vi "Edgertronic-pretrigger_buffer_fill_level.vi"(3 "error in (no error)":errorcluster, 5 "URL":string="192.168.1.101") -> (0 "error out":errorcluster, 1 "Pretrigger Buffer Fill Level:":T1={"Connection Information:"="", "Pretrigger Buffer Fill Level"="20140911165611"}, 2 "Fill Level":i32)   [LabVIEW 2015]
doc: "This VI returns the pretrigger buffer fill level."
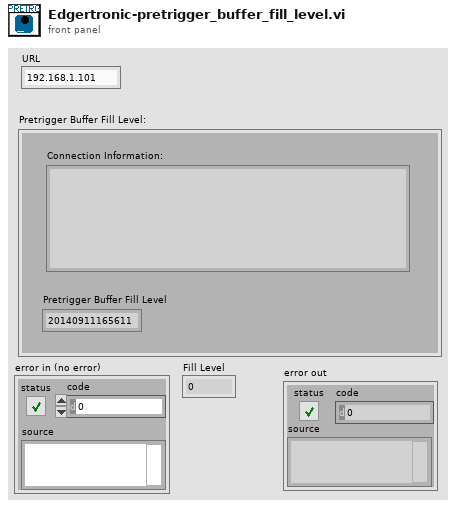
[diagram p1: front panel]
types:
  T1 = cluster{"Connection Information:":string, "Pretrigger Buffer Fill Level":string}
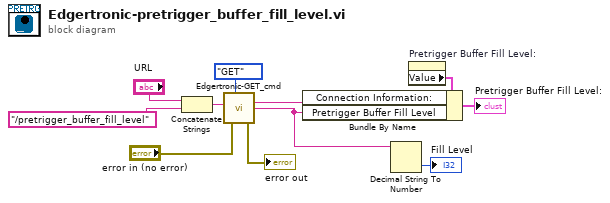
[diagram p0: block diagram]
diagram:
  n1 = Concatenate Strings("URL", "/pretrigger_buffer_fill_level" ("GET Cmd")) -> (w2:string)
  n2 = call "Edgertronic-GET_cmd.vi"("error in (no error)"="error in (no error)", "URL"=w2, "Type"=enum16{"GET", "POST"}."GET") -> ("error out"=→"error out":errorcluster, "data"=w7:string, "Connection Info"=w9:string)  [unwired: 1 in]
  n3 = Decimal String To Number(string=w7) -> (number=→"Fill Level":i32)  [unwired: 2 in, 1 out]
  n4 = property on="Pretrigger Buffer Fill Level:" class="Clust (strict)"() -> ("Value"=w8:T1)  [unwired: 2 in, 2 out]
  n5 = Bundle By Name(cluster=w8, "Connection Information:"=w9, "Pretrigger Buffer Fill Level"=w7) -> (→"Pretrigger Buffer Fill Level:":T1)
